vi "Write Lines.vi"(8 "error in (no error)":errorcluster, 10 "Lines":T1[](array[typedef]), 11 "Scan Engine configuration in":refnum<class "Scan Engine configuration.lvclass">) -> (0 "error out":errorcluster, 3 "Scan Engine configuration out":refnum<class "Scan Engine configuration.lvclass">)   [LabVIEW 2015, in "Scan Engine configuration.lvclass"]
uses:
  Scan Engine configuration.lvclass
  Line.ctl
  <vilib>/NI/Tag Bus Module Framework/channel/TBM channel.lvclass
  Scan Engine configuration.lvclass/Scan Engine configuration.ctl
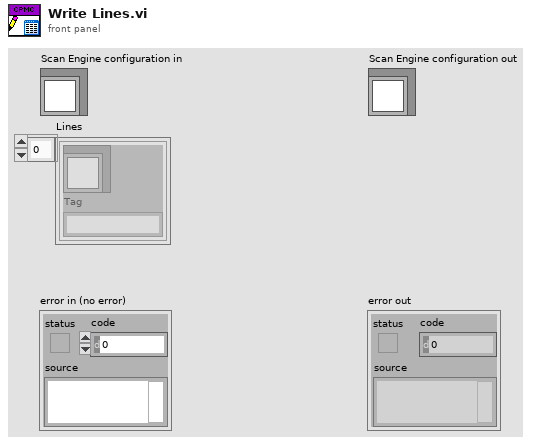
[diagram p1: front panel]
types:
  T1 = typedef "Scan Engine configuration.lvclass/Line.ctl" = cluster{"channel":refnum<class "TBM channel.lvclass">, "Tag":string}
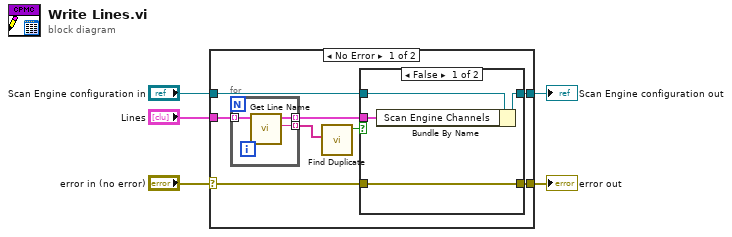
[diagram p0: block diagram]
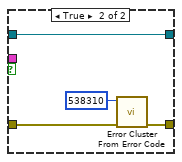
[diagram p2: hidden frame]
diagram:
  n1 = case shown="No Error" "error in (no error)" {
    selector: "error in (no error)" -> [w6 w25]
    tunnel: [w7 w25] -> w4
    tunnel: [w12 w26] -> w2
    tunnel: "Scan Engine configuration in" -> [w13 w26]
    tunnel: "Lines" -> [w11 _]
    frame No Error {
      n2 = for {
        tunnel: w11 -> [w16] mode=indexing
        tunnel: [w15] -> w10 mode=indexing
        tunnel: [w14] -> w9 mode=indexing
        n3 = call "Get Line Name.vi"("Line in"=w16) -> ("Name"=w14:string, "Line out"=w15:T1)  [unwired: 8 in, 1 out]
      }
      n4 = call "Find Duplicate.vi"("Array"=w9) -> ("Duplicate"=w8:bool)  [unwired: 8 in, 2 out]
      n5 = case shown="False" w8 {
        tunnel: w13 -> [w20 w24]
        tunnel: [w19 w24] -> w12
        tunnel: w10 -> [w18 _]
        tunnel: [w17 w22] -> w7
        tunnel: w6 -> [w17 w23]
        frame False {
          n6 = Bundle By Name(cluster=w20, "Scan Engine Channels"=w18) -> (w19:refnum<class "Scan Engine configuration.lvclass">)
        }
        frame True {
          n7 = call <vilib>:"Error Cluster From Error Code.vi"("error in (no error)"=w23, "error code (0)"=538310) -> ("error out"=w22:errorcluster)  [unwired: 7 in]
        }
      }
    }
    frame Error {
    }
  }
  "error out" <- w4
  "Scan Engine configuration out" <- w2
